vi "intakeRoller.vi"() -> ()   [LabVIEW 2018]
uses:
  intakeRoller.ctl
panel:
  in  "speedControl":dbl=0.7
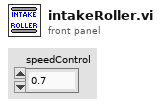
[diagram p1: front panel]
types:
  T1 = typedef "WPI_MotorControlDeviceRef.ctl" = cluster{"DeviceStatus":errorcluster, "Type":T2, "PWM":cluster{"PWM Channel":T3, "DeadBand":T4}, "CAN":cluster{"Device Number":u8, "SetOutput VI Ref":variant, "GetOutput VI Ref":variant, "Enable VI Ref":variant, "Disable VI Ref":variant, "Data":variant}, "Invert":bool, "DIO PWM":cluster{"PWM \"Enable\" Channel":T3, "DIOChannel":T5, "PWM Rate":dbl}}
  T2 = typedef "WPI_MotorControlType.ctl" = enum16{"PWM", "CAN", "DIO PWM"}
  T3 = typedef "FPGA_DIOPWMChannel.ctl" = enum8{"PWM 0", "PWM 1", "PWM 2", "PWM 3", "PWM 4", "PWM 5", "PWM 6", "PWM 7", "PWM 8", "PWM 9", "PWM MXP 0", "PWM MXP 1", "PWM MXP 2", "PWM MXP 3", "PWM MXP 4", "PWM MXP 5", "PWM MXP 6", "PWM MXP 7", "PWM MXP 8", "PWM MXP 9", "Invalid"}
  T4 = typedef "WPI_PWMDeadband.ctl" = cluster{"Name":string, "maxPositivePwm":i32, "minPositivePwm":i32, "centerPwm":i32, "maxNegativePwm":i32, "minNegativePwm":i32, "angularRange":u16}
  T5 = typedef "FPGA_DIOChannel.ctl" = enum8{"DIO 0", "DIO 1", "DIO 2", "DIO 3", "DIO 4", "DIO 5", "DIO 6", "DIO 7", "DIO 8", "DIO 9", "DIO MXP 0", "DIO MXP 1", "DIO MXP 2", "DIO MXP 3", "DIO MXP 4", "DIO MXP 5", "DIO MXP 6", "DIO MXP 7", "DIO MXP 8", "DIO MXP 9", "DIO MXP 10", "DIO MXP 11", "DIO MXP 12", "DIO MXP 13", "DIO MXP 14", "DIO MXP 15", "SPI Port CS1", "SPI Port CS2", "SPI Port CS3", "SPI Port MISO", "SPI Port MOSI", "Invalid"}
  T6 = typedef "intakeRoller.ctl" = enum16{"off", "intake", "outtake"}
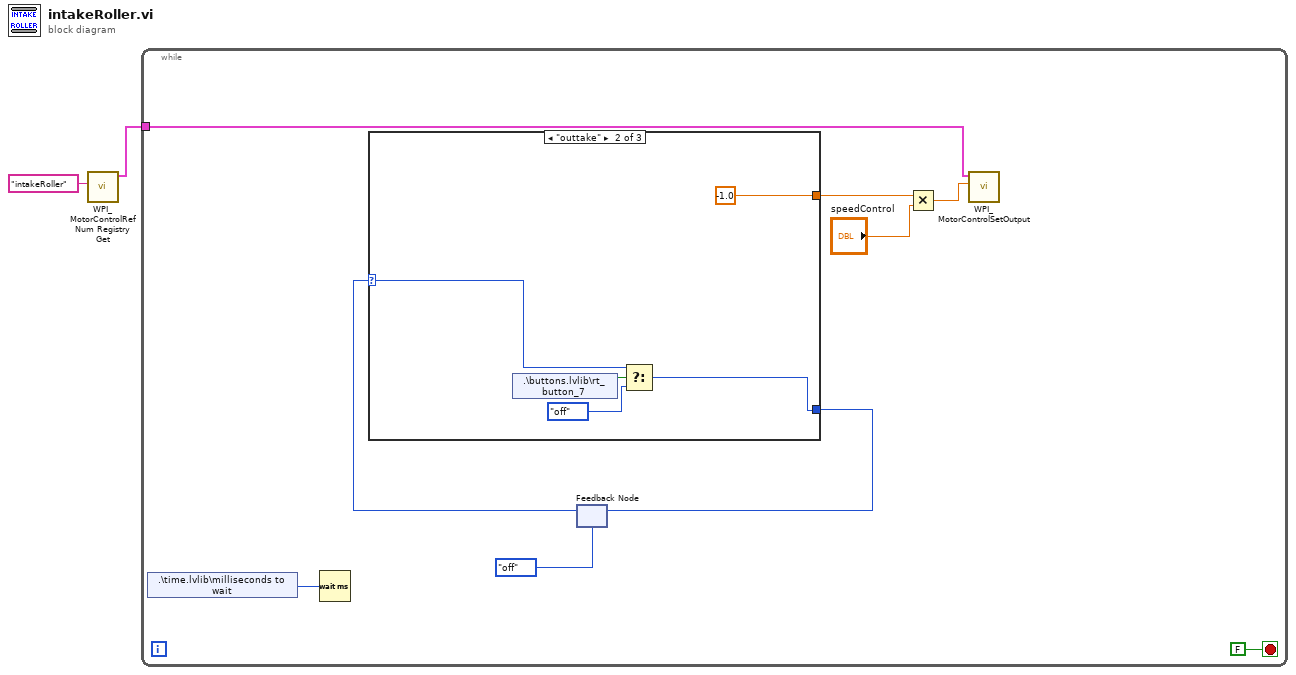
[diagram p0: block diagram]
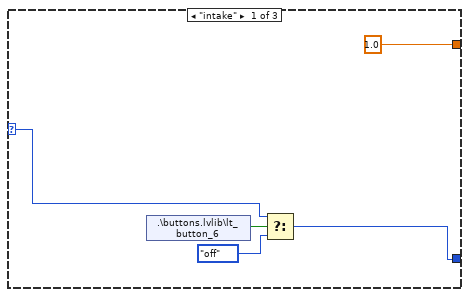
[diagram p2: hidden frame]
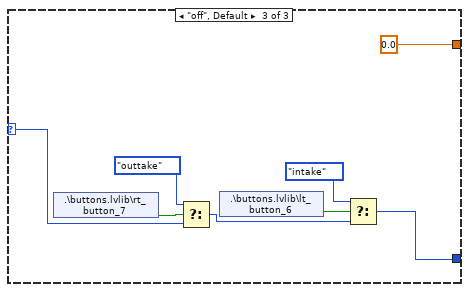
[diagram p3: hidden frame]
diagram:
  n1 = call <vilib>:"WPI_MotorControlRefNum Registry Get.vi"("refnum name"="intakeRoller") -> ("MotorControlDevRef"=w1:T1)  [unwired: 9 in, 1 out]
  n2 = while {
    tunnel: w1 -> [w3]
    stop <- FALSE stop-if-true
    n3 = shared-variable ".\\time.lvlib\\milliseconds to wait"() -> (w8:u32)  [unwired: 1 in, 1 out]
    n4 = Wait (ms)(milliseconds to wait=w8) -> ()  [unwired: 1 out]
    n5 = feedback #1(intakeRoller."off") -> (w9:T6)
    n6 = case shown="\"outtake\"" w9 {
      selector: w9 -> [w14 w20 w29]
      tunnel: [w15 w18 w27] -> w11
      tunnel: [1.0 ("Output") -1.0 ("Output") 0.0 ("Output")] -> w6
      frame "intake" {
        n7 = shared-variable ".\\buttons.lvlib\\lt_button_6"() -> (w16:bool)  [unwired: 1 in, 1 out]
        n8 = Select(t=w14, s=w16, f=intakeRoller."off") -> (s? t:f=w15:T6)
      }
      frame "outtake" {
        n9 = shared-variable ".\\buttons.lvlib\\rt_button_7"() -> (w19:bool)  [unwired: 1 in, 1 out]
        n10 = Select(t=w20, s=w19, f=intakeRoller."off") -> (s? t:f=w18:T6)
      }
      frame "off", Default {
        n11 = shared-variable ".\\buttons.lvlib\\rt_button_7"() -> (w26:bool)  [unwired: 1 in, 1 out]
        n12 = Select(t=intakeRoller."outtake", s=w26, f=w29) -> (s? t:f=w28:T6)
        n13 = shared-variable ".\\buttons.lvlib\\lt_button_6"() -> (w25:bool)  [unwired: 1 in, 1 out]
        n14 = Select(t=intakeRoller."intake", s=w25, f=w28) -> (s? t:f=w27:T6)
      }
    }
    n15 = feedback-in #1(w11) -> ()
    n16 = Multiply(x=w6, y="speedControl") -> (x*y=w5:dbl)
    n17 = call <vilib>:"WPI_MotorControlSetOutput.vi"("Output"=w5, "MotorControlDevRef"=w3) -> ()  [unwired: 7 in, 3 out]
  }
